vi "read_tcx_file _kompuet_lab.vi"(8 "error in":errorcluster, 11 "File Path":path) -> (0 "error out":errorcluster, 2 "Time":timestamp[](array[timestamp]), 3 "Bmp":i32[](array[numeric]))   [LabVIEW 2025]
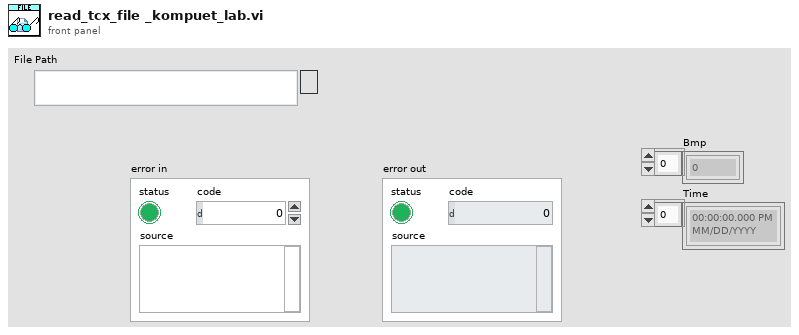
[diagram p1: front panel]
types:
  T1 = enum16{"open", "replace", "create", "open or create", "replace or create", "replace or create with confirmation"}
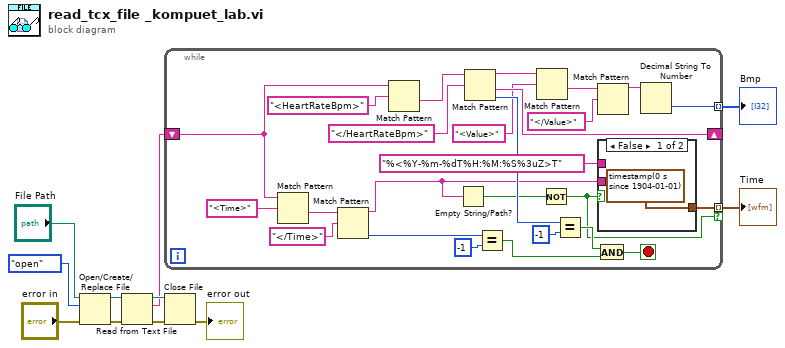
[diagram p0: block diagram]
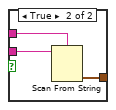
[diagram p2: hidden frame]
diagram:
  n1 = Open/Create/Replace File(file path (use dialog)="File Path", error in="error in", operation (0:open)=T1."open") -> (refnum out=w5:refnum<file>, error out=w9:errorcluster)  [unwired: 3 in, 1 out]
  n2 = Read from Text File(file (use dialog)=w5, error in=w9) -> (refnum out=w4:refnum<file>, text=w3:string, error out=w8:errorcluster)  [unwired: 2 in, 1 out]
  n3 = while {
    shift-right: [w35] -> _
    shift-left: w3 -> [w25]
    tunnel: [w26] -> w2 mode=indexing
    tunnel: [w14] -> w1 mode=indexing if=w13
    stop <- w19 stop-if-true
    n4 = Match Pattern(string=w25, regular expression="<Time>") -> (after substring=w22:string)  [unwired: 1 in, 3 out]
    n5 = Match Pattern(string=w22, regular expression="</Time>") -> (before substring=w12:string, offset past match=w21:i32)  [unwired: 1 in, 2 out]
    n6 = Match Pattern(string=w25, regular expression="<HeartRateBpm>") -> (after substring=w27:string)  [unwired: 1 in, 3 out]
    n7 = Empty String/Path?(string/path=w12) -> (empty?=w16:bool)
    n8 = Match Pattern(string=w27, regular expression="</HeartRateBpm>") -> (before substring=w28:string, after substring=w35:string, offset past match=w34:i32)  [unwired: 1 in, 1 out]
    n9 = Equal?(x=w21, y=-1) -> (x = y?=w17:bool)
    n10 = Match Pattern(string=w28, regular expression="<Value>") -> (after substring=w31:string)  [unwired: 1 in, 3 out]
    n11 = Not(x=w16) -> (.not. x?=w13:bool)
    n12 = Equal?(x=w34, y=-1) -> (x = y?=w18:bool)
    n13 = And(x=w18, y=w17) -> (x .and. y?=w19:bool)
    n14 = Match Pattern(string=w31, regular expression="</Value>") -> (before substring=w29:string)  [unwired: 1 in, 3 out]
    n15 = case shown="False" w13 {
      tunnel: "%<%Y-%m-%dT%H:%M:%S%3uZ>T" ("format string") -> [_ w41]
      tunnel: w12 -> [_ w40]
      tunnel: [timestamp(0 s since 1904-01-01) w39] -> w14
      frame False {
      }
      frame True {
        n16 = Scan From String(format string=w41, input string=w40) -> (output 1=w39:timestamp)  [unwired: 3 in, 3 out]
      }
    }
    n17 = Decimal String To Number(string=w29) -> (number=w26:i32)  [unwired: 2 in, 1 out]
  }
  "Bmp" <- w2
  "Time" <- w1
  n18 = Close File(refnum=w4, error in=w8) -> (error out=→"error out":errorcluster)  [unwired: 1 out]
